vi "led_pulse.vi"() -> ()   [LabVIEW 2014]
uses:
  <vilib>/DAQmx/write.llb/DAQmx Write (Digital Bool 1Line 1Point).vi
  <vilib>/DAQmx/create/channels.llb/DAQmx Create Channel (DO-Digital Output).vi
  <vilib>/DAQmx/miscellaneous.llb/DAQmx Fill In Error Info.vi
panel:
  out "Boolean":bool
  in  "stop":bool
  in  "Lines":tag="Dev1/port0/line0:7"
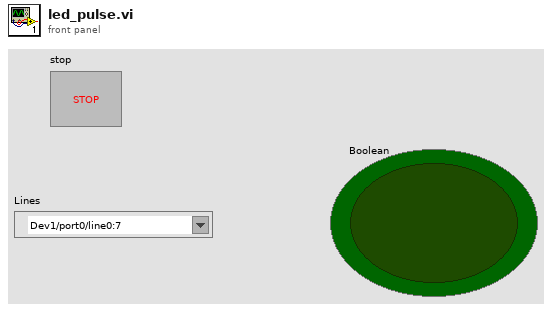
[diagram p1: front panel]
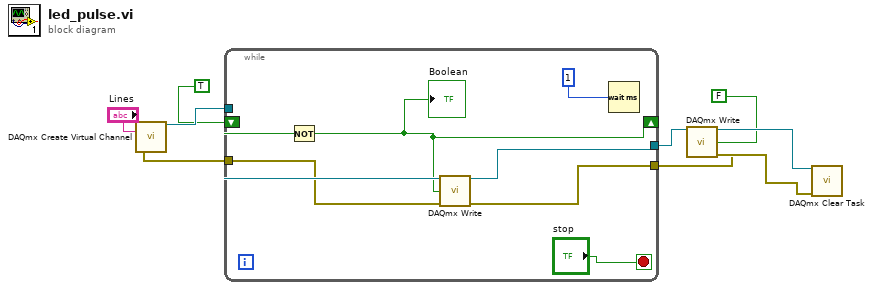
[diagram p0: block diagram]
diagram:
  n1 = call-poly <vilib>:"DAQmx Create Virtual Channel.vi"("lines"="Lines") -> ("task out"=w4:refnum<k21>, "error out"=w3:errorcluster)  [unwired: 13 in]
  n2 = while {
    tunnel: [w16] -> w6
    tunnel: [w15] -> w5
    tunnel: w4 -> [w14]
    tunnel: w3 -> [w13]
    shift-right: [w10] -> _
    shift-left: TRUE -> [w12]
    stop <- "stop" stop-if-true
    n3 = Not(x=w12) -> (.not. x?=w10:bool)
    "Boolean" <- w10
    n4 = call-poly <vilib>:"DAQmx Write.vi"("task/channels in"=w14, "data"=w10, "error in"=w13) -> ("task out"=w16:refnum<k21>, "error out"=w15:errorcluster)  [unwired: 10 in, 1 out]
    n5 = Wait (ms)(milliseconds to wait=u32 1 ("millisecond timer value")) -> ()  [unwired: 1 out]
  }
  n6 = call-poly <vilib>:"DAQmx Write.vi"("task/channels in"=w6, "data"=FALSE, "error in"=w5) -> ("task out"=w8:refnum<k21>, "error out"=w7:errorcluster)  [unwired: 10 in, 1 out]
  n7 = call <vilib>:"DAQmx Clear Task.vi"("task in"=w8, "error in"=w7) -> ()  [unwired: 13 in, 1 out]
